vi "StrQueue-Insert (string).vi"(2 "queue in":string[](array[string]), 4 "string":string) -> (5 "queue out":string[](array[string]))   [LabVIEW 2015]
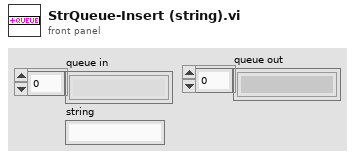
[diagram p1: front panel]
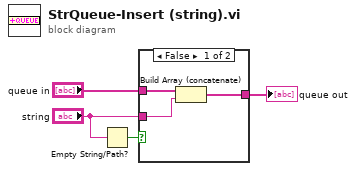
[diagram p0: block diagram]
diagram:
  n1 = Empty String/Path?(string/path="string") -> (empty?=w1:bool)
  n2 = case shown="False" w1 {
    tunnel: "queue in" -> [w7 w8]
    tunnel: "string" -> [w6 _]
    tunnel: [w5 w8] -> w3
    frame False {
      n3 = Build Array (concatenate)(w7, w6) -> (w5:string[])
    }
    frame True {
    }
  }
  "queue out" <- w3
